vi "kloehn_pump_command.vi"(7 "wait for ready to return?":bool=TRUE, 10 "Send String":string, 11 "kloehn session in":T1={"VISA resource out"="COM12", "error out"={"status"=FALSE, "code"=0, "source"=""}}) -> (1 "Unparsed Response String":string, 2 "Parsed Response String":string, 3 "kloehn session out":T1={"VISA resource out"="COM12", "error out"={"status"=FALSE, "code"=0, "source"=""}}, 5 "Status":enum16{"Ready", "Busy"}(ring))   [LabVIEW 2010]
panel:
  # "This VI differs from the regular Kloehn read and write VI in that if a pump command is being issed (that is, to have the pump actually do something), this VI gives you the option of waiting for ready status before passing along control of the program. This makes it easier to string along pump commands which would otherwise conflict with eachother. Waiting should be the default - you can pass no if you you want to continue program flow and don't have any soon pending pump commands to issue."
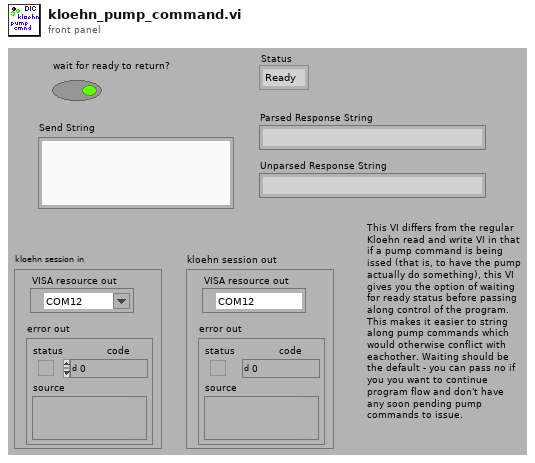
[diagram p1: front panel]
types:
  T1 = cluster{"VISA resource out":refnum<visa-resource-name>, "error out":errorcluster}
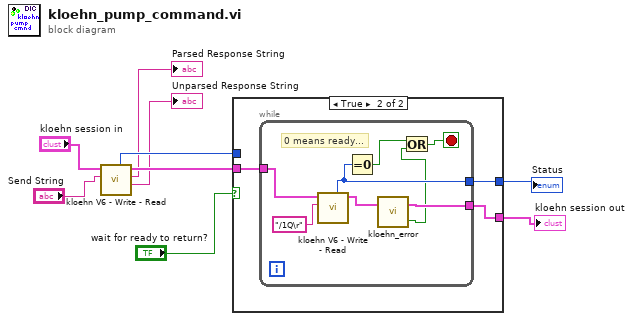
[diagram p0: block diagram]
diagram:
  n1 = call "kloehn V6 - Write - Read.vi"("Send String"="Send String", "kloehn session in"="kloehn session in") -> ("Unparsed Response String"=→"Unparsed Response String":string, "Parsed Response String"=→"Parsed Response String":string, "kloehn session out"=w4:T1, "Status"=w6:enum16{"Ready", "Busy"})  [unwired: 6 in]
  n2 = case shown="True" "wait for ready to return?" {
    tunnel: w6 -> [w11 _]
    tunnel: [w11 w13] -> w5
    tunnel: w4 -> [w10 w14]
    tunnel: [w10 w12] -> w3
    frame False {
    }
    frame True {
      n3 = while {
        tunnel: w14 -> [w21]
        tunnel: [w20] -> w13
        tunnel: [w18] -> w12
        stop <- w15 stop-if-true
        # "0 means ready..."
        n4 = call "kloehn V6 - Write - Read.vi"("Send String"="/1Q\r", "kloehn session in"=w21) -> ("kloehn session out"=w19:T1, "Status"=w20:enum16{"Ready", "Busy"})  [unwired: 6 in, 2 out]
        n5 = Equal To 0?(x=w20) -> (x = 0?=w16:bool)
        n6 = call "kloehn_error.vi"("kloehn session in"=w19) -> ("error?"=w17:bool, "kloehn session out"=w18:T1)  [unwired: 1 in]
        n7 = Or(x=w16, y=w17) -> (x .or. y?=w15:bool)
      }
    }
  }
  "Status" <- w5
  "kloehn session out" <- w3
